vi "Rpm_To_Feet_Per_Sec.vi"(10 "RPM":dbl, 11 "Diameter":dbl) -> (3 "Numeric":dbl)   [LabVIEW 2020]
doc: "A simple VI that Allows for an easy conversion from RPM to FT/S base on input RPM and Wheel Diameter in inches"
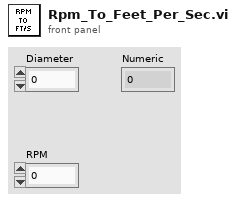
[diagram p1: front panel]
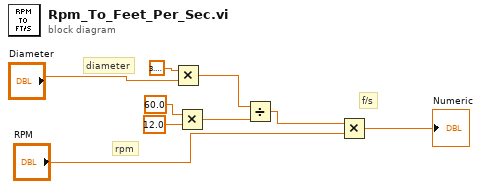
[diagram p0: block diagram]
diagram:
  # "f/s"
  # "diameter"
  # "rpm"
  n1 = Multiply(x=3.141592653589793, y="Diameter") -> (x*y=w6:dbl)
  n2 = Multiply(x=60.0, y=12.0) -> (x*y=w3:dbl)
  n3 = Divide(x=w6, y=w3) -> (x/y=w7:dbl)
  n4 = Multiply(x=w7, y="RPM") -> (x*y=→"Numeric":dbl)
